vi "algo.test.vi"(9 "reset":bool, 10 "debug":bool) -> ()   [LabVIEW 2022 SP3]
uses:
  <vilib>/Platform/TimedLoop/XDataNode/XDataNode.xnode
  <vilib>/Platform/TimedLoop/XDataNode/nitl_modes.ctl
  <vilib>/Platform/TimedLoop/XDataNode/XDNodeRunTimeDep.lvlib
  <vilib>/Platform/TimedLoop/XDataNode/wakeup.ctl
  <vilib>/Platform/TimedLoop/XDataNode/timing_clust.ctl
  <vilib>/rvi/DataTransferAndStorage/Container/XNode/niFpgaContainer.xnode
  <vilib>/rvi/interface/RandomDataEmulation/nirviRandomDataFpgaMultiElementTemplate.vi
  <vilib>/rvi/FIFO/Fifo_Resource/nirvififoEmulationRead.vi
  common/orderbook.command.type.ctl
  common/orderbook.command.ctl
  <vilib>/rvi/FIFO/Fifo_Resource/nirvififoEmulationWrite.vi
  <vilib>/rvi/interface/RandomDataEmulation/nirviRandomDataFpgaReadWriteTemplate.vi
  types/algo.val.watchlist.ctl
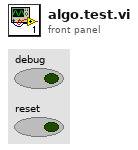
[diagram p1: front panel]
types:
  T1 = typedef "XDNodeRunTimeDep.lvlib/timing_clust.ctl" = cluster{"Expected End [f-1]":u64, "Actual End [f-1]":u64, "Finished Late? [f-1]":bool, "Expected End [i-1]":u64, "Actual End [i-1]":u64, "Finished Late? [i-1]":bool, "Expected Start [i]":u64, "Actual Start [i]":u64, "Expected Start [f]":u64, "Actual Start [f]":u64, "Source Name":string, "Structure Name":string, "Period":i64, "Deadline":i64, "Offset":i64, "Start":i64, "Priority":i32, "Timeout":i32, "Mode":T2, "Wakeup Reason":T3, "Error":errorcluster, "Source Type":string, "Secondary Source Type":string, "Global End Time":u64, "Global Start Time":u64, "Frame Duration":u64, "Iteration Duration":u64, "Assigned CPU":i32, "I/O Scan Engine Mode":u32}
  T2 = typedef "XDNodeRunTimeDep.lvlib/nitl_modes.ctl" = enum32{"No Change", "Process missed periods, maintain original phase", "Discard missed periods, maintain original phase", "Process missed periods, ignore original phase", "Discard missed periods, ignore original phase"}
  T3 = typedef "XDNodeRunTimeDep.lvlib/wakeup.ctl" = enum32{"Normal", "Aborted", "Asynchronous wakeup", "Timing source error", "Timed loop error", "Timeout"}
  T4 = typedef "orderbook.command.ctl" = cluster{"type":T5, "side":u8, "orderId ":u64, "quantity":u32, "symbol":u64, "price":u64, "executed.qty":u32, "canceled.qty":u32, "remaining.qty":u32, "seconds":u64, "nanoseconds":u64}
  T5 = typedef "orderbook.command.type.ctl" = enum8{"Time", "AddOrder", "OrderExecuted", "OrderExecutedAtPrice", "ReduceSize", "ModifyOrder", "DeleteOrder", "Get.State", "Get.All.Orders", "Get.Top"}
  T6 = typedef "algo.val.watchlist.ctl" = cluster{"symbol":u64, "buy.size":u16, "buy.start.addr":u16, "sell.start.addr":u16, "sell.size":u16, "min.ask":u32, "max.bid":u32}
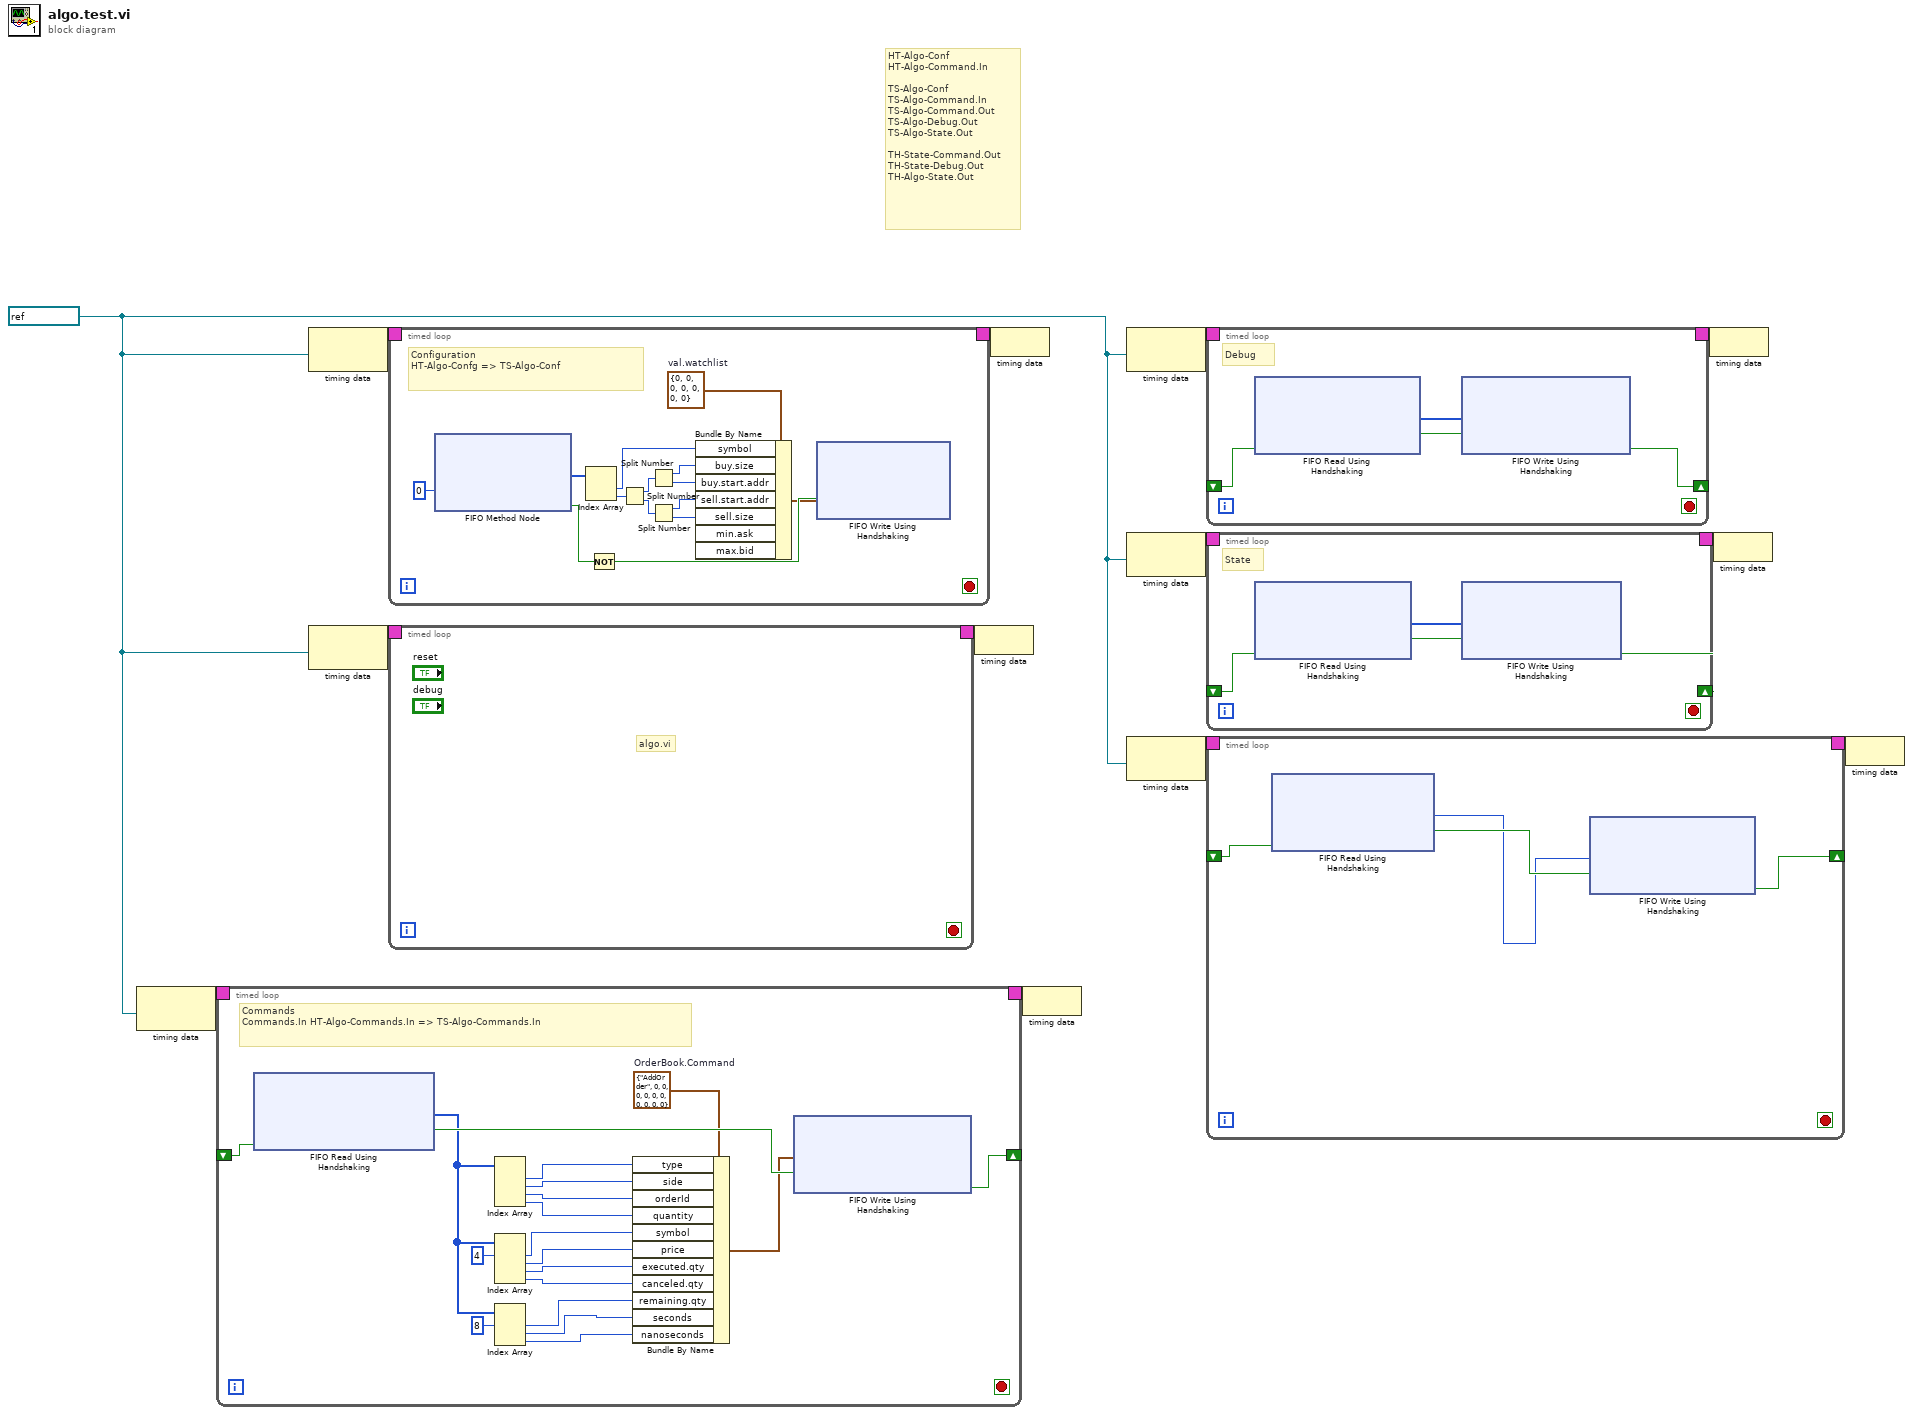
[diagram p0: block diagram]
diagram:
  w1 = refnum<k21> "160MHz" ("Source Name")
  # "HT-Algo-Conf\nHT-Algo-Command.In\n\nTS-Algo-Conf\nTS-Algo-Command.In\nTS-Algo-Command.Out\nTS-Algo-Debug.Out\nTS-Algo-State.Out\n\nTH-State-Command.Out\nTH-State-Debug.Out\nTH-Algo-State.Out"
  n1 = node-c288(w1) -> (w7:T1)
  n2 = timed-loop {
    timing: w7 -> [_]
    timing-out: [_] -> w6
    shift-right: [w32] -> _
    shift-left: _ -> [w31]
    stop <- _ stop-if-true
    w29 = T4 {"type"=enum."AddOrder", "side"=0, "orderId "=0, "quantity"=0, "symbol"=0, "price"=0, "executed.qty"=0, "canceled.qty"=0, "remaining.qty"=0, "seconds"=0, "nanoseconds"=0}  # OrderBook.Command
    # "Commands\nCommands.In HT-Algo-Commands.In => TS-Algo-Commands.In"
    n3 = xnode ("FIFO Read Using Handshaking")("Ready for Output"=w31) -> ("Element"=w27:u64[], "Output Valid"=w30:bool)  [unwired: 1 in, 1 out]
    n4 = Index Array(array=w27) -> (element #1=w24:u64, element #2=w23:u64, element #3=w22:u64, element #4=w21:u64)  [unwired: 4 in]
    n5 = Index Array(array=w27, index #1=4 ("index")) -> (element #1=w20:u64, element #2=w19:u64, element #3=w18:u64, element #4=w17:u64)  [unwired: 3 in]
    n6 = Index Array(array=w27, index #1=8 ("index")) -> (element #1=w16:u64, element #2=w15:u64, element #3=w14:u64)  [unwired: 2 in]
    n7 = Bundle By Name(cluster=w29, "type"=w24, "side"=w23, "orderId"=w22, "quantity"=w21, "symbol"=w20, "price"=w19, "executed.qty"=w18, "canceled.qty"=w17, "remaining.qty"=w16, "seconds"=w15, "nanoseconds"=w14) -> (w28:T4)
    n8 = xnode ("FIFO Write Using Handshaking")("Element"=w28, "Input Valid"=w30) -> ("Ready for Input"=w32:bool)  [unwired: 1 in, 1 out]
  }
  n9 = node-c288(w1) -> (w11:T1)
  n10 = node-c288(w1) -> (w13:T1)
  n11 = timed-loop {
    timing: w11 -> [_]
    timing-out: [_] -> w10
    stop <- _ stop-if-true
    w35 = T6 {"symbol"=0, "buy.size"=0, "buy.start.addr"=0, "sell.start.addr"=0, "sell.size"=0, "min.ask"=0, "max.bid"=0}  # val.watchlist
    # "Configuration\nHT-Algo-Confg => TS-Algo-Conf"
    n12 = xnode ("FIFO Method Node")("Timeout"=0) -> ("Element"=w45:u64[], "Timed Out?"=w47:bool)  [unwired: 1 in, 1 out]
    n13 = Index Array(array=w45) -> (element #1=w44:u64, element #2=w43:u64)  [unwired: 2 in]
    n14 = Not(x=w47) -> (.not. x?=w46:bool)
    n15 = Split Number(x=w43) -> (hi(x)=w41:u32, lo(x)=w42:u32)
    n16 = Split Number(x=w41) -> (hi(x)=w40:u16, lo(x)=w39:u16)
    n17 = Split Number(x=w42) -> (hi(x)=w37:u16, lo(x)=w38:u16)
    n18 = Bundle By Name(cluster=w35, "symbol"=w44, "buy.size"=w40, "buy.start.addr"=w39, "sell.start.addr"=w37, "sell.size"=w38) -> (w36:T6)  [unwired: 2 in]
    n19 = xnode ("FIFO Write Using Handshaking")("Element"=w36, "Input Valid"=w46) -> ()  [unwired: 1 in, 2 out]
  }
  n20 = timed-loop {
    timing: w13 -> [_]
    timing-out: [_] -> w12
    stop <- _ stop-if-true
    # "algo.vi"
  }
  n21 = node-c288(w12) -> ()
  n22 = node-c288(w10) -> ()
  n23 = node-c288(w6) -> ()
  n24 = node-c288(w1) -> (w9:T1)
  n25 = node-c288(w1) -> (w3:T1)
  n26 = node-c288(w1) -> (w5:T1)
  n27 = timed-loop {
    timing: w9 -> [_]
    timing-out: [_] -> w8
    shift-right: [w56] -> _
    shift-left: _ -> [w55]
    stop <- _ stop-if-true
    # "Debug"
    n28 = xnode ("FIFO Read Using Handshaking")("Ready for Output"=w55) -> ("Element"=w53:u64[], "Output Valid"=w54:bool)  [unwired: 1 in, 1 out]
    n29 = xnode ("FIFO Write Using Handshaking")("Element"=w53, "Input Valid"=w54) -> ("Ready for Input"=w56:bool)  [unwired: 1 in, 1 out]
  }
  n30 = timed-loop {
    timing: w3 -> [_]
    timing-out: [_] -> w2
    shift-right: [w62] -> _
    shift-left: _ -> [w61]
    stop <- _ stop-if-true
    # "State"
    n31 = xnode ("FIFO Read Using Handshaking")("Ready for Output"=w61) -> ("Element"=w59:u64[], "Output Valid"=w60:bool)  [unwired: 1 in, 1 out]
    n32 = xnode ("FIFO Write Using Handshaking")("Element"=w59, "Input Valid"=w60) -> ("Ready for Input"=w62:bool)  [unwired: 1 in, 1 out]
  }
  n33 = timed-loop {
    timing: w5 -> [_]
    timing-out: [_] -> w4
    shift-right: [w68] -> _
    shift-left: _ -> [w67]
    stop <- _ stop-if-true
    n34 = xnode ("FIFO Read Using Handshaking")("Ready for Output"=w67) -> ("Element"=w65:u64, "Output Valid"=w66:bool)  [unwired: 1 in, 1 out]
    n35 = xnode ("FIFO Write Using Handshaking")("Element"=w65, "Input Valid"=w66) -> ("Ready for Input"=w68:bool)  [unwired: 1 in, 1 out]
  }
  n36 = node-c288(w8) -> ()
  n37 = node-c288(w2) -> ()
  n38 = node-c288(w4) -> ()
